vi "Pockels Cal-Outer structure.vi"(0 "Number of objectives + 1":i32, 1 "Skip cal for all remaining objectives?":bool, 5 "Objective's name":string, 9 "Parent FOR loop's index":i32, 12 "Pockels calibration voltage steps sequence":dbl[](array[numeric]), 14 "Voltage %":u16[](array[numeric])) -> (4 "Skip cal for all remaining objectives":bool, 6 "Results array":string[](array[string]), 8 "Cancel & Exit":bool, 10 "Timed out or errored out":bool, 15 "error out":errorcluster)   [LabVIEW 2013]
uses:
  Globals/gl_Calibration globals.vi
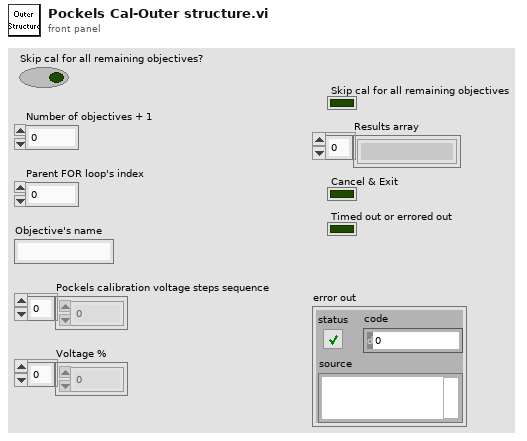
[diagram p1: front panel]
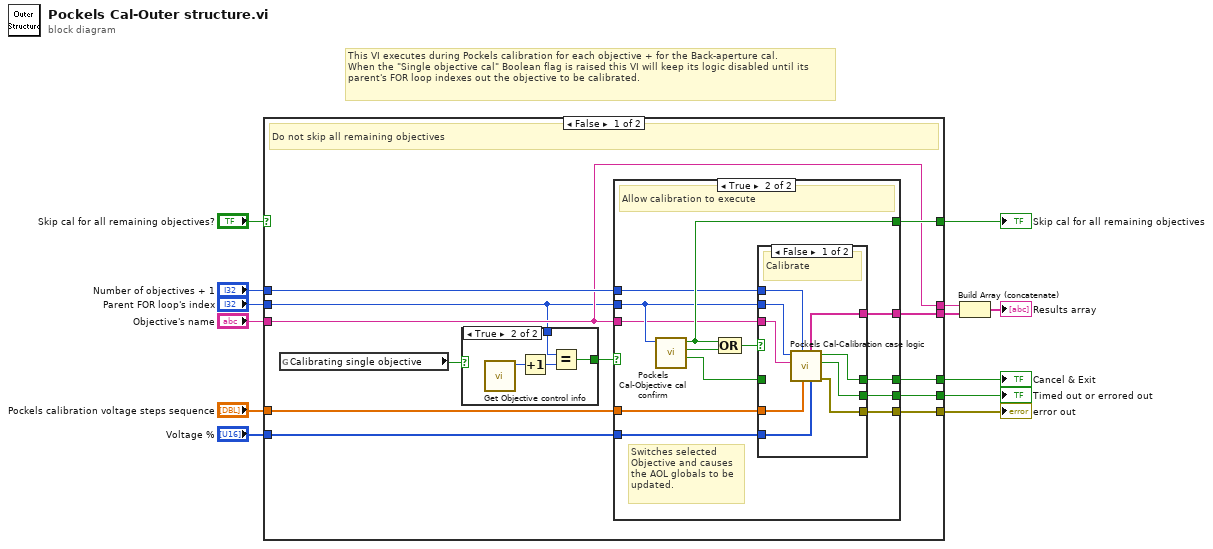
[diagram p0: block diagram]
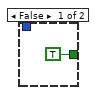
[diagram p2: hidden frame]
diagram:
  # "This VI executes during Pockels calibration for each objective + for the Back-aperture cal.\nWhen the \"Single objective cal\" Boolean flag is raised this VI will keep its logic disabled until its parent's FOR loop indexes out the objective to be calibrated."
  n1 = case shown="False" "Skip cal for all remaining objectives?" {
    selector: "Skip cal for all remaining objectives?" -> [_ w55]
    tunnel: [w24 _] -> w1
    tunnel: [w23 _] -> w3
    tunnel: [w22 _] -> w4
    tunnel: "Number of objectives + 1" -> [w21 _]
    tunnel: "Parent FOR loop's index" -> [w16 _]
    tunnel: [w20 _] -> w7
    tunnel: "Objective's name" -> [w17 w54]
    tunnel: "Pockels calibration voltage steps sequence" -> [w19 _]
    tunnel: "Voltage %" -> [w18 _]
    tunnel: [w25 w55] -> w10
    tunnel: [w17 w54] -> w13
    frame False {
      # "Do not skip all remaining objectives"
      n2 = global read "gl_Calibration globals.vi" "Calibrating single objective"() -> (w15:bool)
      n3 = case shown="True" w15 {
        tunnel: w16 -> [_ w28]
        tunnel: [TRUE w27] -> w14
        frame False {
        }
        frame True {
          n4 = call "Get Objective control info.vi"() -> ("Selection index"=w30:i32)  [unwired: 7 in, 4 out]
          n5 = Increment(x=w30) -> (x+1=w29:i32)
          n6 = Equal?(x=w28, y=w29) -> (x = y?=w27:bool)
        }
      }
      n7 = case shown="True" w14 {
        tunnel: [_ w43] -> w25
        tunnel: [_ w42] -> w24
        tunnel: [_ w41] -> w23
        tunnel: [_ w40] -> w22
        tunnel: w21 -> [_ w39]
        tunnel: w16 -> [_ w38]
        tunnel: [_ w37] -> w20
        tunnel: w19 -> [_ w36]
        tunnel: w18 -> [_ w35]
        tunnel: w17 -> [_ w32]
        frame False {
          # "Do not execute calibration"
        }
        frame True {
          # "Switches selected Objective and causes the AOL globals to be updated."
          # "Allow calibration to execute"
          n8 = call "Pockels Cal-Objective cal confirm.vi"("Index of current outer loop iteraton"=w38) -> ("Cancelled"=w31:bool, "Skip cal for this objective"=w34:bool, "Skip cal for all objectives"=w43:bool)  [unwired: 7 in, 1 out]
          n9 = Compound Arithmetic op=OR(w43, w34) -> (w33:bool)
          n10 = case shown="False" w33 {
            tunnel: [w44 _] -> w42
            tunnel: [w52 w53] -> w41
            tunnel: [w51 _] -> w40
            tunnel: w39 -> [w50 _]
            tunnel: w38 -> [w49 _]
            tunnel: [w48 _] -> w37
            tunnel: w32 -> [w47 _]
            tunnel: w36 -> [w46 _]
            tunnel: w35 -> [w45 _]
            tunnel: w31 -> [_ w53]
            frame False {
              # "Calibrate"
              n11 = call "Pockels Cal-Calibration case logic.vi"("Voltage %"=w45, "Pockels calibration voltage steps sequence"=w46, "Number of objectives + 1"=w50, "Objective's name"=w47, "Parent FOR loop's index"=w49) -> ("error out"=w48:errorcluster, "Timed out or errored out"=w51:bool, "Cancel & Exit"=w52:bool, "Output Strings"=w44:string[])  [unwired: 3 in]
            }
            frame True {
              # "Calibration for this objective was skipped"
              # "Skipped"
            }
          }
        }
      }
    }
    frame True {
      # "Skips all additional objective calibrations"
      # "Skip cal for all remaining objectives"
    }
  }
  "Skip cal for all remaining objectives" <- w10
  "error out" <- w7
  "Timed out or errored out" <- w4
  "Cancel & Exit" <- w3
  n12 = Build Array (concatenate)(w13, w1) -> (→"Results array":string[])
